vi "Get_Tree_Item_Source_Contained_File.vi"(8 "error in (no error)":errorcluster, 11 "IB_TreeCtrFileItem in":refnum<class "IB_Tree_Item_Source_Contained_File.lvclass">) -> (0 "error out":errorcluster, 2 "data":T1, 3 "IB_TreeCtrFileItem out":refnum<class "IB_Tree_Item_Source_Contained_File.lvclass">)   [LabVIEW 2020, in "IB_Tree_Item_Source_Contained_File.lvclass"]
uses:
  <vilib>/AppBuilder/IB_Classes/Tree_Item_Source_Contained_File/IB_Tree_Item_Source_Contained_File.lvclass
  <vilib>/AppBuilder/IB_Classes/Tree_Item_Source_Contained_File/IB_Tree_Item_Source_Contained_File.lvclass/IB_Tree_Item_Source_Contained_File.ctl
  <vilib>/AppBuilder/IB_Classes/Tree_Item_Virtual_Folder/IB_Tree_Item_Virtual_Folder.lvclass
  <vilib>/AppBuilder/IB_Classes/Tree_Item_Source_Contained_File/IB_Tree_Item_Source_Contained_File.ctl
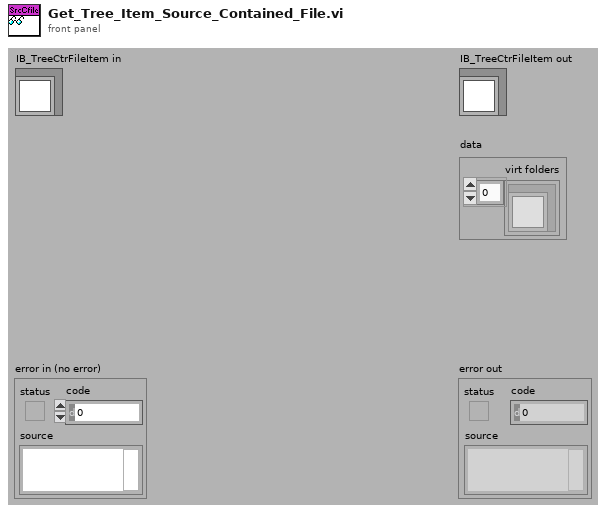
[diagram p1: front panel]
types:
  T1 = typedef "IB_Tree_Item_Source_Contained_File.ctl" = cluster{"virt folders":refnum<class "IB_Tree_Item_Virtual_Folder.lvclass">[]}
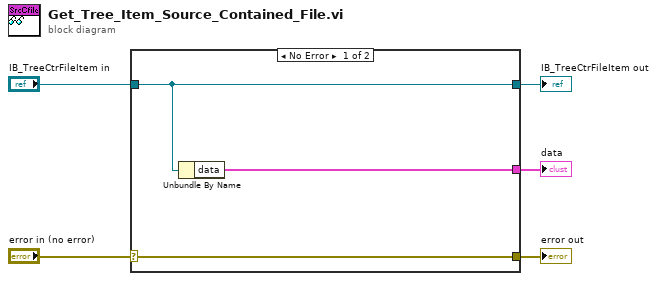
[diagram p0: block diagram]
diagram:
  n1 = case shown="No Error" "error in (no error)" {
    selector: "error in (no error)" -> [w8 w9]
    tunnel: [w8 w9] -> w4
    tunnel: [w7 w10] -> w2
    tunnel: "IB_TreeCtrFileItem in" -> [w7 w10]
    tunnel: [w6 _] -> w1
    frame No Error {
      n2 = Unbundle By Name(w7) -> ("data"=w6:T1)
    }
    frame Error {
    }
  }
  "error out" <- w4
  "IB_TreeCtrFileItem out" <- w2
  "data" <- w1
